vi "DIO In.vi"(1 "Number of Inputs":i32=1 min=1 max=10, 2 "Mode":enum8{"Start", "Run", "Finish"}(ring)) -> (0 "Values":bool[](array[boolean]))   [LabVIEW 2014]
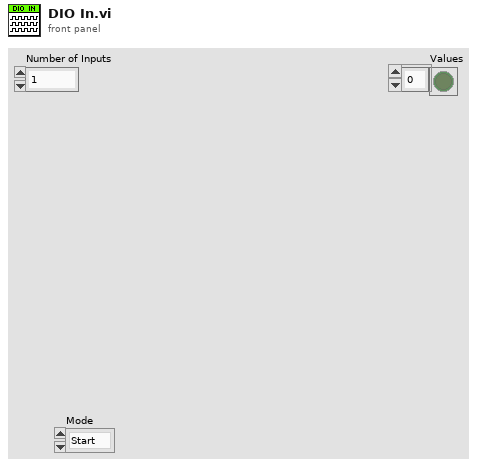
[diagram p1: front panel]
types:
  T1 = typedef "WPI_DigitalInputDevRef.ctl" = cluster{"DevStatus":errorcluster, "DIO Channel":T2, "Controller":T3}
  T2 = typedef "FPGA_DIOChannel.ctl" = enum8{"DIO 0", "DIO 1", "DIO 2", "DIO 3", "DIO 4", "DIO 5", "DIO 6", "DIO 7", "DIO 8", "DIO 9", "DIO MXP 0", "DIO MXP 1", "DIO MXP 2", "DIO MXP 3", "DIO MXP 4", "DIO MXP 5", "DIO MXP 6", "DIO MXP 7", "DIO MXP 8", "DIO MXP 9", "DIO MXP 10", "DIO MXP 11", "DIO MXP 12", "DIO MXP 13", "DIO MXP 14", "DIO MXP 15", "Invalid"}
  T3 = typedef "FPGA_TypedefDigitalModule.ctl" = enum16{"Controller 1"}
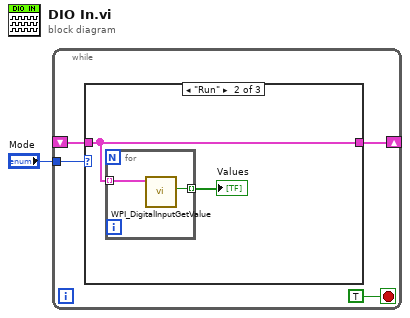
[diagram p0: block diagram]
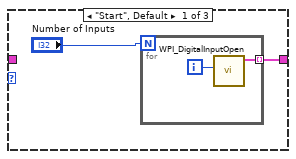
[diagram p2: hidden frame]
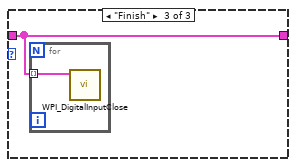
[diagram p3: hidden frame]
diagram:
  n1 = while {
    tunnel: "Mode" -> [w5]
    shift-right: [w4] -> _
    shift-left: _ -> [w3]
    stop <- TRUE stop-if-true
    n2 = case shown="\"Run\"" w5 {
      tunnel: [w6 w11 w14] -> w4
      tunnel: w3 -> [_ w11 w14]
      frame "Start", Default {
        n3 = for {
          N: "Number of Inputs" -> [_]
          tunnel: [w8] -> w6 mode=indexing
          i -> [w9]
          n4 = call <vilib>:"WPI_DigitalInputOpen.vi"("DIO Channel"=w9) -> ("DigitalInputDevRef"=w8:T1)  [unwired: 9 in, 1 out]
        }
      }
      frame "Run" {
        n5 = for {
          tunnel: w11 -> [w13] mode=indexing
          tunnel: [w12] -> w10 mode=indexing
          n6 = call <vilib>:"WPI_DigitalInputGetValue.vi"("DigitalInputDevRef"=w13) -> ("Value"=w12:bool)  [unwired: 8 in, 2 out]
        }
        "Values" <- w10
      }
      frame "Finish" {
        n7 = for {
          tunnel: w14 -> [w15] mode=indexing
          n8 = call <vilib>:"WPI_DigitalInputClose.vi"("DigitalInputDevRef"=w15) -> ()  [unwired: 10 in, 1 out]
        }
      }
    }
  }
